vi "init_scope_data_Qs.vi"(2 "max queue size (-1, unlimited)":i32=1) -> (0 "scope Q data":T1)   [LabVIEW 2023]
panel:
  in  "output cluster":T1
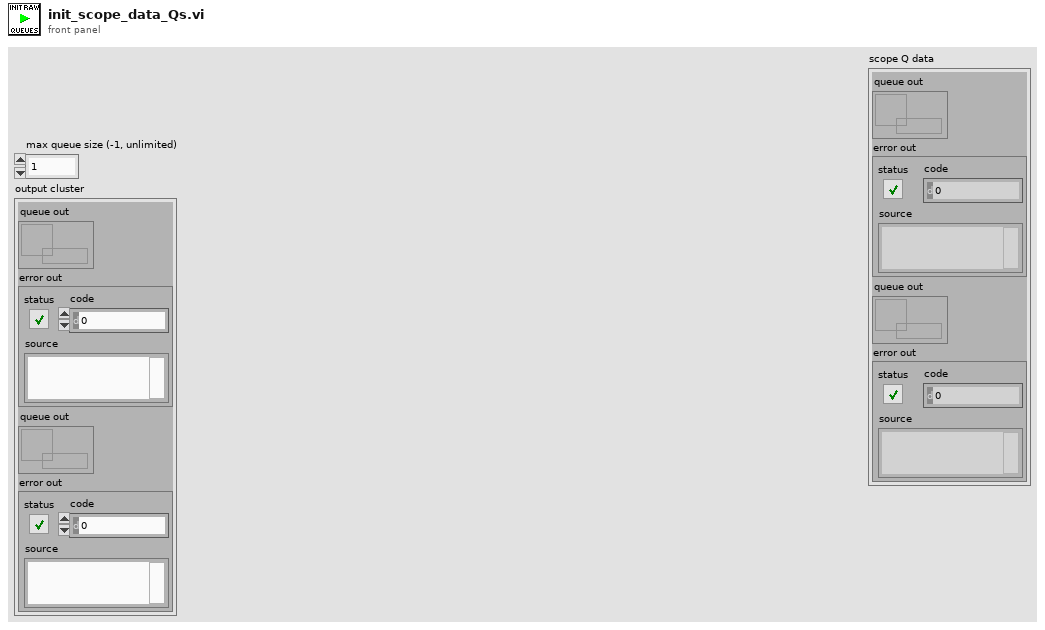
[diagram p1: front panel]
types:
  T1 = cluster{"queue out":refnum<queue>, "error out":errorcluster, "queue out":refnum<queue>, "error out":errorcluster}
  T2 = cluster{"wfm info":cluster{"actualSamples":i32, "absoluteInitialX":dbl, "relativeInitialX":dbl, "xIncrement":dbl, "offset":dbl, "gain":dbl, "reserved1":dbl, "reserved2":dbl}, "Offset WFm":waveform(dbl), bool}
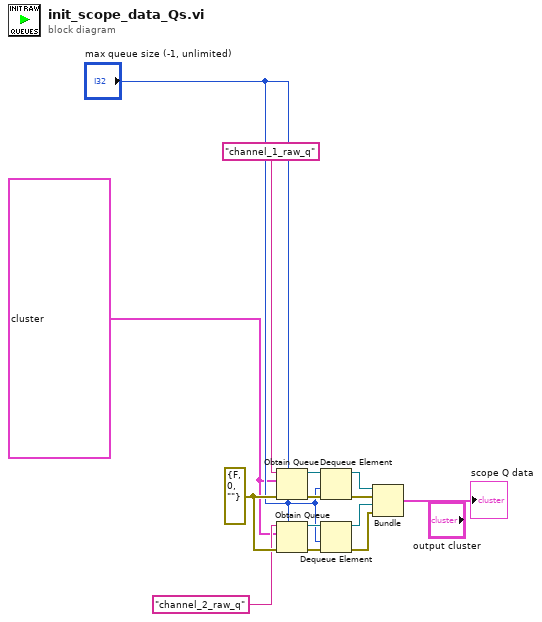
[diagram p0: block diagram]
diagram:
  w2 = T2 {"wfm info"={"actualSamples"=0, "absoluteInitialX"=0.0, "relativeInitialX"=0.0, "xIncrement"=0.0, "offset"=0.0, "gain"=0.0, "reserved1"=0.0, "reserved2"=0.0}, "Offset WFm"={"t0"=timestamp(0 s since 1904-01-01), "dt"=1.0, "Y"=[]}, FALSE} ("output cluster")
  w9 = errorcluster {"status"=FALSE, "code"=0, "source"=""} ("error in (no error)")
  n1 = Obtain Queue(max queue size (-1, unlimited)="max queue size (-1, unlimited)", name (unnamed)="channel_1_raw_q" ("Q1 Name"), element data type=w2, error in (no error)=w9) -> (queue out=w14:refnum<queue>, error out=w13:errorcluster)  [unwired: 1 in, 1 out]
  n2 = Obtain Queue(max queue size (-1, unlimited)="max queue size (-1, unlimited)", name (unnamed)="channel_2_raw_q" ("Q2 Name"), element data type=w2, error in (no error)=w9) -> (queue out=w12:refnum<queue>, error out=w11:errorcluster)  [unwired: 1 in, 1 out]
  n3 = Dequeue Element(queue=w14, timeout in ms (-1)="max queue size (-1, unlimited)", error in (no error)=w13) -> (queue out=w7:refnum<queue>, error out=w6:errorcluster)  [unwired: 2 out]
  n4 = Dequeue Element(queue=w12, timeout in ms (-1)="max queue size (-1, unlimited)", error in (no error)=w11) -> (queue out=w5:refnum<queue>, error out=w4:errorcluster)  [unwired: 2 out]
  n5 = Bundle("queue out"=w7, "error out"=w6, "queue out"=w5, "error out"=w4) -> (→"scope Q data":T1)  [unwired: 1 in]
